vi "Intan_mainControlPanel_64chan.vi"() -> ()   [LabVIEW 2017]
panel:
  out "Serial Port Type":string
  out "DT samp (us)":dbl
  out "ADC calib":bool
  in  "Config Hardware Filter":bool=TRUE
  in  "Start Data Stream":bool
  out "HeaderFilePath":path
  in  "Save Display Data":bool
  in  "ConfigReg [0:7, aPwr]":bool=TRUE
  out "Config Result":string
  out "Teensy response":string
  out "actual fs (Hz)":dbl
  out "Raw data file path":path
  in  "Save Raw Data":bool=TRUE
  in  "Desired Fs (Hz)":u16=200
  in  "VISA resource name":refnum<visa-resource-name>="COM33"
  in  "R_L source":u8(ring)=1 items=["ON-chip", "OFF-chip"]
  in  "Lower cutoff":u8(ring)=12 items=["10 Hz", "7.5 Hz", "5.0 Hz", "3.0 Hz", "2.5 Hz", "2.0 Hz", "1.5 Hz", "1.0 Hz", "0.75 Hz", "0.5 Hz", "0.3 Hz", "0.25 Hz", "0.10 Hz"]
  in  "Upper cutoff":u8(ring)=12 items=["5.0 kHz", "3.0 kHz", "2.5 kHz", "2.0 kHz", "1.5 kHz", "1.0 kHz", "750 Hz", "500 Hz", "300 Hz", "250 Hz", "200 Hz", "150 Hz", "100 Hz"]
  # "Intan-Teensy Bioelectric Module: configure hardware and serial port 64 chan"
  # "Configure all settings, then click run arrow.\n\nWhen config is complete, click the purple\nbutton to start data stream.\n\nSeparate VI will pop open to display signals"
  # "TODO 01 May 2017 JE\n\nSTATUS: Operational, beta.\n\nSOFTWARE issues:\n\n - Set decimation ratio to ensure Nsamps in display never exceeds chart limit\nor sensible human visibility bound (for now set chart history length = 50000.\nFor typical max sampling rates of 500 Hz in our applications, this still allows up to 100 s\nof data display (ridiculously long).  In practice, could probably increase performance\nby decreasing chart history to something smaller like 20000.\n\n\n- Make bdf style header and write to file (low priority)\n\n -  Stream to main fig window, Present only does this in subVI (IntanStream_Parallel Loops.vi)\n  SOLN: just pop open subVI automatically when called, but pre-set filters (?)\n\nHARDWARE issues: \n\n\nNeed to gracefully recover when data sync is lost. Option to reboot Teensy and recover connection? \nCurrent error checking not working, don' know why.  Software reset tricky to implement:\nhttps://forum.pjrc.com/archive/index.php/t-24304.html\nBest solution for now, unplug then replug power.  This puts Teensy back into initial state.\n\n-Option to stream subset of channels.  This will allow higher data rate for wireless streaming, if desired."
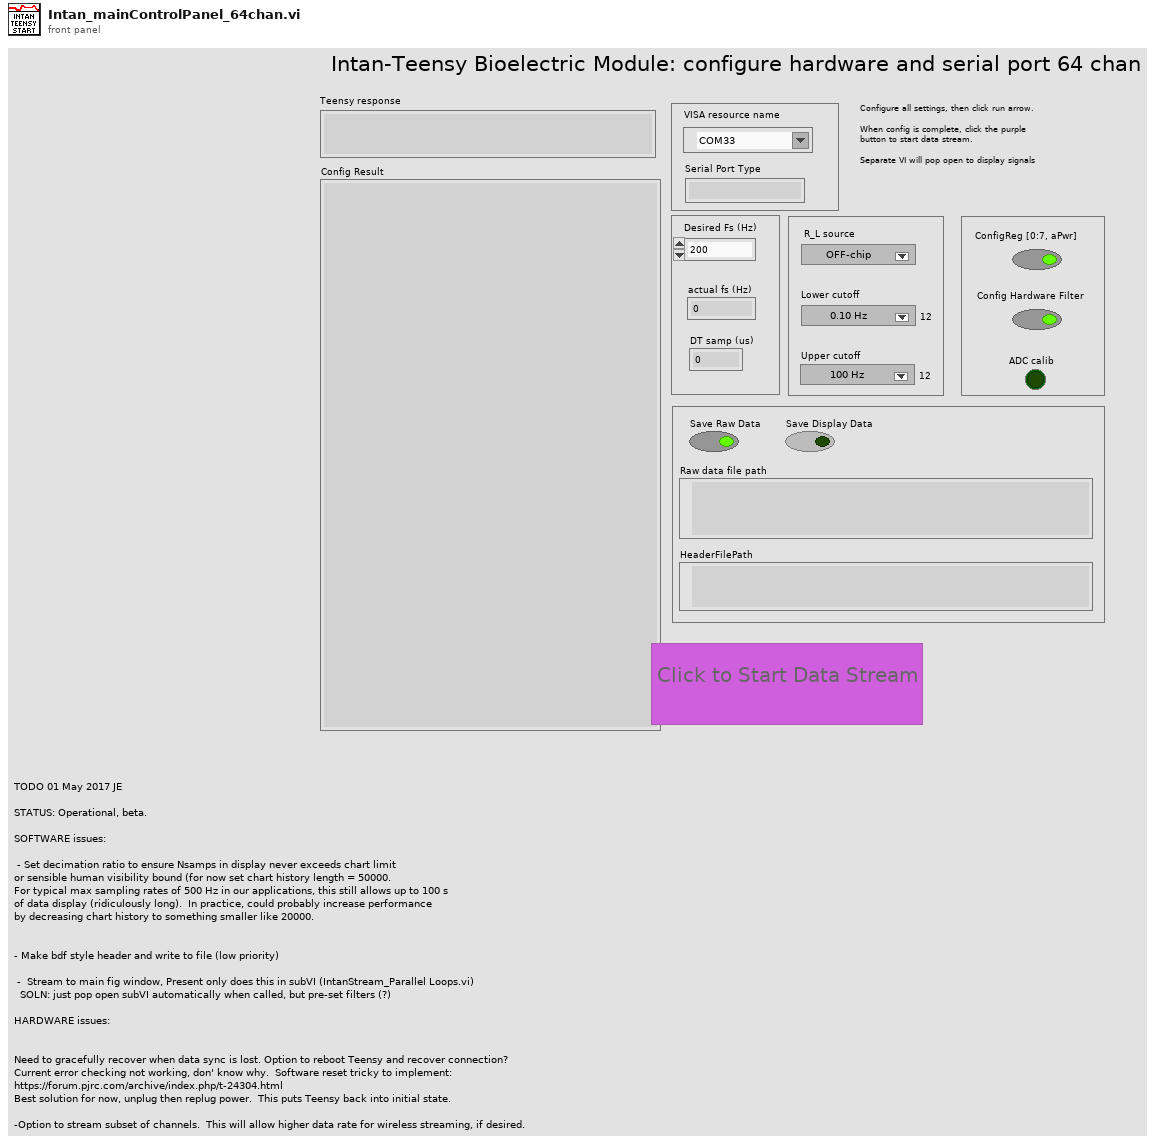
[diagram p1: front panel]
types:
  T1 = enum8{"Enabled", "Disabled", "Disabled and Grayed Out"}
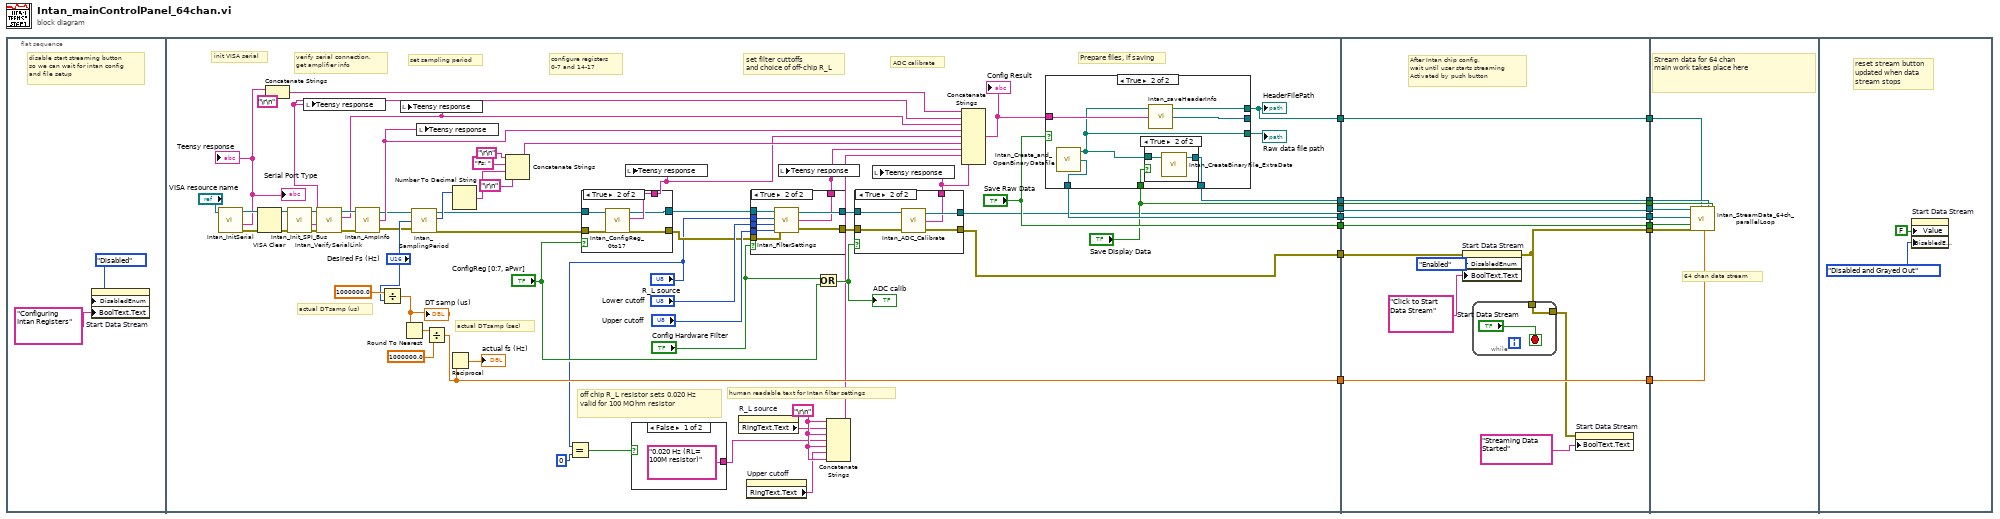
[diagram p0: block diagram]
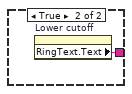
[diagram p2: hidden frame]
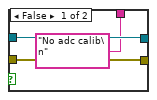
[diagram p3: hidden frame]
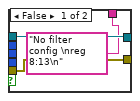
[diagram p4: hidden frame]
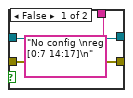
[diagram p5: hidden frame]
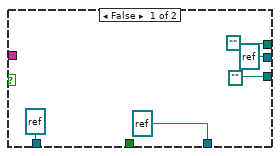
[diagram p6: hidden frame]
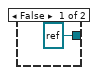
[diagram p7: hidden frame]
diagram:
  n1 = flat-sequence {
    tunnel: [w74] -> w10
    tunnel: [w62] -> w9
    tunnel: [w59] -> w8
    tunnel: ["Save Raw Data"] -> w7
    tunnel: ["Save Display Data"] -> w6
    tunnel: [w45] -> w5
    tunnel: [w44] -> w3
    tunnel: [w38] -> w1
    tunnel: [w130] -> w16
    tunnel: [w136] -> w15
    tunnel: [w135] -> w14
    tunnel: [w134] -> w13
    tunnel: [w133] -> w12
    tunnel: [w132] -> w11
    tunnel: w6 -> [w132]
    tunnel: w7 -> [w133]
    tunnel: w8 -> [w134]
    tunnel: w9 -> [w135]
    tunnel: w10 -> [w136]
    tunnel: w5 -> [w129]
    tunnel: [w128] -> w4
    tunnel: w3 -> [w128]
    tunnel: [w127] -> w2
    tunnel: w1 -> [w127]
    tunnel: w16 -> [w143]
    tunnel: w15 -> [w141]
    tunnel: w14 -> [w146]
    tunnel: w13 -> [w144]
    tunnel: w12 -> [w142]
    tunnel: w11 -> [w145]
    tunnel: w4 -> [w140]
    tunnel: w2 -> [w139]
    frame #0 {
      # "disable start streaming button\nso we can wait for intan config\nand file setup"
      n2 = property on="Start Data Stream" class="Bool (strict)"("DisabledEnum"=T1."Disabled" ("Disabled"), "BoolText.Text"="Configuring Intan Registers" ("Boolean Text.Text")) -> ()  [unwired: 2 in, 2 out]
    }
    frame #1 {
      w33 = "\r\n"
      # "off chip R_L resistor sets 0.020 Hz \nvalid for 100 MOhm resistor"
      # "human readable text for Intan filter settings"
      # "Prepare files, if saving"
      # "ADC calibrate"
      # "set filter cuttoffs \nand choice of off-chip R_L"
      # "configure registers\n0-7 and 14-17"
      # "set sampling period"
      # "verify serial connection,\nget amplifier info"
      # "init VISA serial"
      # "actual DTsamp (sec)"
      # "actual DTsamp (us)"
      n3 = call "Intan_InitSerial.vi"("VISA resource name"="VISA resource name") -> ("VISA resource name out"=w37:refnum<visa-resource-name>, "Text response"=w35:string, "error out"=w73:errorcluster)  [unwired: 3 in]
      "Teensy response" <- w35
      "Serial Port Type" <- w35
      n4 = VISA Clear(VISA resource name=w37, error in (no error)=w73) -> (VISA resource name out=w24:refnum<visa-resource-name>, error out=w23:errorcluster)
      n5 = Concatenate Strings(w35, "\r\n") -> (w20:string)
      n6 = call "Intan_Init_SPI_Bus.vi"("error in"=w23, "VISA resource name"=w24) -> ("error out"=w22:errorcluster, "Text response"=w19:string, "VISA resource name out"=w21:refnum<visa-resource-name>)  [unwired: 3 in]
      n7 = local write "Teensy response"(w19) -> ()
      n8 = call "Intan_VerifySerialLink.vi"("error in"=w22, "VISA resource name"=w21) -> ("error out"=w75:errorcluster, "Text response"=w71:string, "VISA resource name out"=w76:refnum<visa-resource-name>)  [unwired: 7 in]
      n9 = call "Intan_AmpInfo.vi"("error in"=w75, "VISA resource name"=w76) -> ("error out"=w55:errorcluster, "Text response"=w72:string, "VISA resource name out"=w56:refnum<visa-resource-name>)  [unwired: 1 in]
      n10 = Divide(x=1000000.0, y="Desired Fs (Hz)") -> (x/y=w39:dbl)
      "DT samp (us)" <- w39
      n11 = local write "Teensy response"(w71) -> ()
      n12 = Round To Nearest(number=w39) -> (nearest integer value=w64:dbl)
      n13 = call "Intan_SamplingPeriod.vi"("VISA resource name"=w56, "Desired Fs (Hz)"="Desired Fs (Hz)", "error in"=w55) -> ("VISA resource name out"=w54:refnum<visa-resource-name>, "FS actual (Hz)"=w70:i32, "error out"=w53:errorcluster)  [unwired: 1 out]
      n14 = local write "Teensy response"(w72) -> ()
      n15 = Divide(x=w64, y=1000000.0 ("x")) -> (x/y=w62:dbl)
      n16 = Reciprocal(x=w62) -> (1/x=→"actual fs (Hz)":dbl)
      n17 = Number To Decimal String(number=w70) -> (decimal integer string=w69:string)  [unwired: 1 in]
      n18 = Concatenate Strings("\r\n", "Fs: " ("string"), w69, "\r\n") -> (w67:string)
      n19 = Equal?(x="R_L source", y=u8 0) -> (x = y?=w28:bool)
      n20 = case shown="True" "ConfigReg [0:7, aPwr]" {
        tunnel: w54 -> [w102 w108]
        tunnel: w53 -> [w101 w107]
        tunnel: ["No config \nreg [0:7 14:17]\n" ("Text response") w106] -> w52
        tunnel: [w102 w105] -> w49
        tunnel: [w101 w104] -> w48
        frame False {
        }
        frame True {
          n21 = call "Intan_ConfigReg_0to17.vi"("error in"=w107, "VISA resource name"=w108) -> ("error out"=w104:errorcluster, "Text response"=w106:string, "VISA resource name out"=w105:refnum<visa-resource-name>)  [unwired: 7 in]
        }
      }
      n22 = local write "Teensy response"(w52) -> ()
      n23 = case shown="False" w28 {
        tunnel: ["0.020 Hz (RL= 100M resistor)" ("string") w81] -> w26
        frame False {
        }
        frame True {
          n24 = property on="Lower cutoff" class="Ring (strict)"() -> ("RingText.Text"=w81:string)  [unwired: 2 in, 2 out]
        }
      }
      n25 = property on="R_L source" class="Ring (strict)"() -> ("RingText.Text"=w31:string)  [unwired: 2 in, 2 out]
      n26 = property on="Upper cutoff" class="Ring (strict)"() -> ("RingText.Text"=w32:string)  [unwired: 2 in, 2 out]
      n27 = case shown="True" "Config Hardware Filter" {
        tunnel: "R_L source" -> [_ w100]
        tunnel: "Lower cutoff" -> [_ w99]
        tunnel: "Upper cutoff" -> [_ w98]
        tunnel: w49 -> [w92 w97]
        tunnel: w48 -> [w91 w96]
        tunnel: [w92 w95] -> w47
        tunnel: [w91 w94] -> w46
        tunnel: ["No filter config \nreg 8:13\n" ("Text response") w93] -> w43
        frame False {
        }
        frame True {
          n28 = call "Intan_FilterSettings.vi"("VISA resource name"=w97, "R_L source"=w100, "Lower cutoff"=w99, "Upper cutoff"=w98, "error in"=w96) -> ("VISA resource name out"=w95:refnum<visa-resource-name>, "Text response"=w93:string, "error out"=w94:errorcluster)
        }
      }
      n29 = local write "Teensy response"(w43) -> ()
      n30 = Or(x="Config Hardware Filter", y="ConfigReg [0:7, aPwr]") -> (x .or. y?=w42:bool)
      "ADC calib" <- w42
      n31 = Concatenate Strings(w33, w31, w33, w26, w33, w32, w33) -> (w29:string)
      n32 = case shown="True" w42 {
        tunnel: w47 -> [w84 w89]
        tunnel: w46 -> [w83 w88]
        tunnel: [w83 w87] -> w45
        tunnel: [w84 w86] -> w44
        tunnel: ["No adc calib\n" ("Text response") w85] -> w30
        frame False {
        }
        frame True {
          n33 = call "Intan_ADC_Calibrate.vi"("error in"=w88, "VISA resource name"=w89) -> ("error out"=w87:errorcluster, "Text response"=w85:string, "VISA resource name out"=w86:refnum<visa-resource-name>)  [unwired: 1 in]
        }
      }
      n34 = local write "Teensy response"(w30) -> ()
      n35 = Concatenate Strings(w20, w19, w71, w72, w52, w67, w43, w29, w30) -> (w60:string)
      "Config Result" <- w60
      n36 = case shown="True" "Save Raw Data" {
        tunnel: [refnum<file> refnum ("refnum out") w120] -> w74
        tunnel: w60 -> [_ w119]
        tunnel: [refnum<file> refnum ("refnum out") w118] -> w59
        tunnel: "Save Display Data" -> [_ w117]
        tunnel: [path "" w116] -> w38
        tunnel: [path "" w115] -> w50
        tunnel: [refnum<file> refnum ("hdr_file_ref_num_out") w114] -> _
        frame False {
        }
        frame True {
          n37 = call "Intan_Create_and_OpenBinaryDatafile.vi"() -> ("file path"=w115:path, "refnum out"=w120:refnum<file>)  [unwired: 2 in, 1 out]
          n38 = case shown="True" w117 {
            tunnel: w115 -> [_ w123]
            tunnel: [refnum<file> refnum ("refnum out") w122] -> w118
            frame False {
            }
            frame True {
              n39 = call "Intan_CreateBinaryFile_ExtraData.vi"("DataFilePath"=w123) -> ("refnum out"=w122:refnum<file>)  [unwired: 3 in, 1 out]
            }
          }
          n40 = call "Intan_saveHeaderInfo.vi"("header text"=w119, "DataFilePath"=w115) -> ("hdr_file_ref_num_out"=w114:refnum<file>, "HeaderFilePath"=w116:path)  [unwired: 1 in, 1 out]
        }
      }
      "HeaderFilePath" <- w38
      "Raw data file path" <- w50
    }
    frame #2 {
      # "After Intan chip config,\nwait until user starts streaming\nActivated by push button"
      n41 = property on="Start Data Stream" class="Bool (strict)"(error in=w129, "DisabledEnum"=T1."Enabled" ("Disabled"), "BoolText.Text"="Click to Start Data Stream" ("Boolean Text.Text")) -> (error out=w130:errorcluster)  [unwired: 1 in, 1 out]
      n42 = while {
        tunnel: w130 -> [w137]
        tunnel: [w137] -> w125
        stop <- "Start Data Stream" stop-if-true
      }
      n43 = property on="Start Data Stream" class="Bool (strict)"(error in=w125, "BoolText.Text"="Streaming Data Started" ("Boolean Text.Text")) -> ()  [unwired: 1 in, 2 out]
    }
    frame #3 {
      # "64 chan data stream"
      # "Stream data for 64 chan\nmain work takes place here"
      n44 = call "Intan_StreamData_64ch_parallelLoop.vi"("VISA resource name"=w140, "refnum in"=w141, "Save Binary Data"=w142, "error in"=w143, "hdr fpath"=w139, "DT_scale (sec)"=w146, "aux file ref num"=w144, "save aux file"=w145) -> ()  [unwired: 8 in, 4 out]
    }
    frame #4 {
      # "reset stream button \nupdated when data\nstream stops"
      n45 = property on="Start Data Stream" class="Bool (strict)"("Value"=FALSE ("Start Data Stream"), "DisabledEnum"=T1."Disabled and Grayed Out" ("Disabled")) -> ()  [unwired: 2 in, 2 out]
    }
  }
